vi "escribir_puertoserie.vi"(0 "buffer in":string, 1 "dato A":i32, 2 "dato B":i32, 3 "dato C":i32, 4 "dato D":i32, 5 "dato E":i32, 6 "fin de cadena 2":string=" S", 7 "ENVIAR":bool) -> (20 "buffer out":string, 24 "serial write":string, 27 "Cadena a enviar":string)   [LabVIEW 2017]
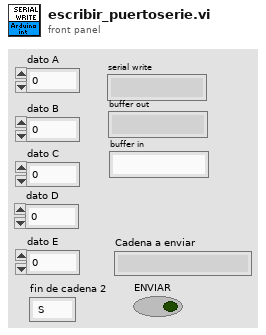
[diagram p1: front panel]
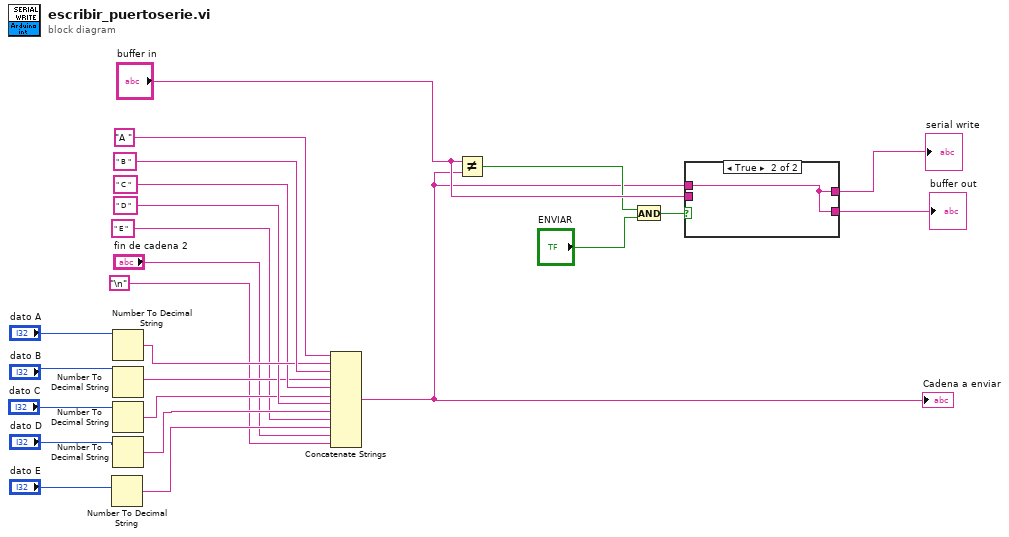
[diagram p0: block diagram]
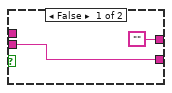
[diagram p2: hidden frame]
diagram:
  n1 = Number To Decimal String(number="dato E") -> (decimal integer string=w5:string)  [unwired: 1 in]
  n2 = Number To Decimal String(number="dato A") -> (decimal integer string=w17:string)  [unwired: 1 in]
  n3 = Number To Decimal String(number="dato B") -> (decimal integer string=w11:string)  [unwired: 1 in]
  n4 = Number To Decimal String(number="dato C") -> (decimal integer string=w10:string)  [unwired: 1 in]
  n5 = Number To Decimal String(number="dato D") -> (decimal integer string=w9:string)  [unwired: 1 in]
  n6 = Concatenate Strings("A " ("string"), w17, " B " ("string"), w11, " C " ("string"), w10, " D " ("string"), w9, " E " ("string"), w5, "fin de cadena 2", "\n") -> (w1:string)
  "Cadena a enviar" <- w1
  n7 = Not Equal?(x="buffer in", y=w1) -> (x != y?=w20:bool)
  n8 = And(x=w20, y="ENVIAR") -> (x .and. y?=w19:bool)
  n9 = case shown="True" w19 {
    tunnel: ["" w27] -> w23
    tunnel: [w25 w27] -> w21
    tunnel: "buffer in" -> [w25 _]
    tunnel: w1 -> [_ w27]
    frame False {
    }
    frame True {
    }
  }
  "serial write" <- w23
  "buffer out" <- w21
